vi "当前实验模式.vi"() -> ()   [LabVIEW 2013]
panel:
  in  "当前实验模式":string
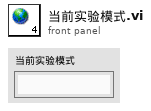
[diagram p1: front panel]
diagram:
